vi "prova 2.vi"() -> ()   [LabVIEW 2021]
panel:
  in  "index":dbl
  out "value":dbl
  out "size(s)":i32
  out "Array 3":dbl[](array[slide]) scale=0.0..10.0
  out "Array 4":bool[](array[boolean])
  in  "Array 2":bool[](array[boolean])
  in  "Array":dbl[](array[numeric])
  out "Waveform Graph":dbl[](graph)
  out "Waveform Chart":dbl(graph)
  in  "stop":bool
  in  "Boolean 3":bool
  out "String 2":string
  out "Integer2":dbl
  in  "Integer":dbl
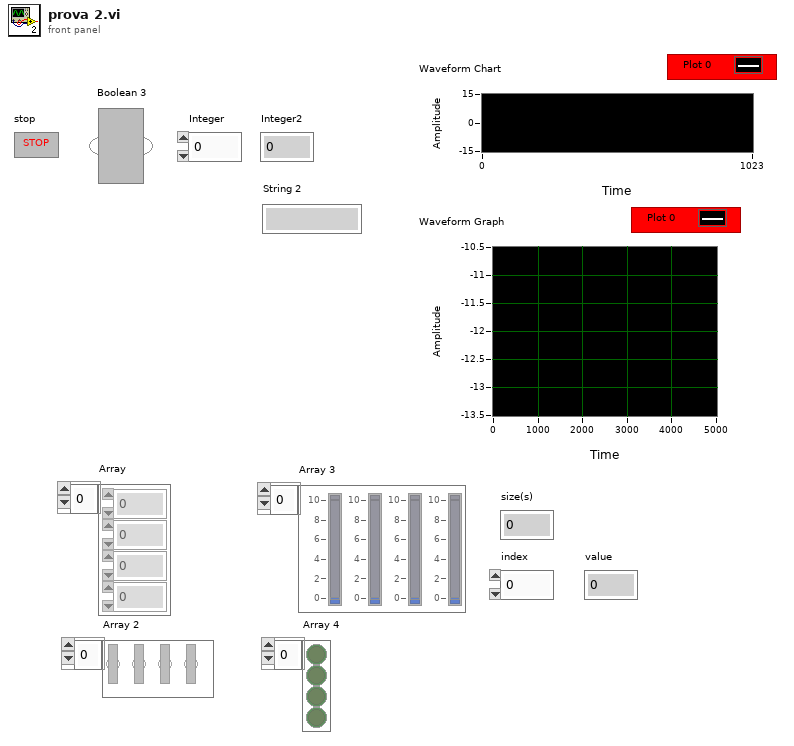
[diagram p1: front panel]
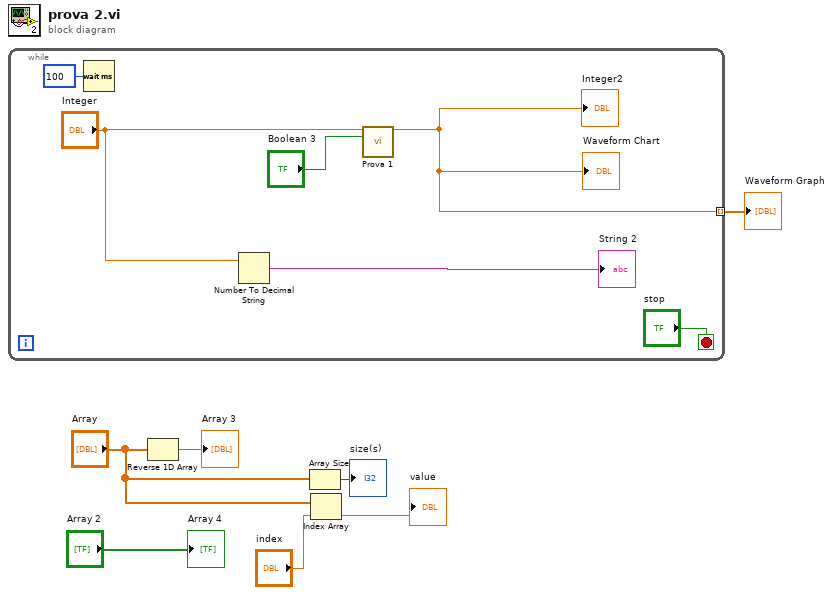
[diagram p0: block diagram]
diagram:
  n1 = while {
    tunnel: [w8] -> w7 mode=indexing
    stop <- "stop" stop-if-true
    n2 = Wait (ms)(milliseconds to wait=u32 100) -> ()  [unwired: 1 out]
    n3 = Number To Decimal String(number="Integer") -> (decimal integer string=→"String 2":string)  [unwired: 1 in]
    n4 = call "Prova 1.vi"("Integer"="Integer", "Boolean"="Boolean 3") -> ("Numeric"=w8:dbl)  [unwired: 13 in]
    "Integer2" <- w8
    "Waveform Chart" <- w8
  }
  "Waveform Graph" <- w7
  n5 = Reverse 1D Array(array="Array") -> (reversed array=→"Array 3":dbl[])
  n6 = Array Size(array="Array") -> (size(s)=→"size(s)":i32)
  n7 = Index Array(array="Array", index="index") -> (element=→"value":dbl)
  "Array 4" <- "Array 2"
